vi "constellation_SubVI_-1.vi"(10 "Array":dbl[][](array[numeric]), 11 "N":dbl) -> (3 "Cluster":cluster{dbl[], dbl[]})   [LabVIEW 2014]
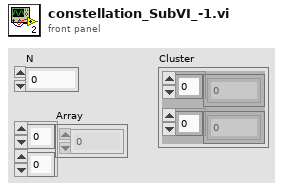
[diagram p1: front panel]
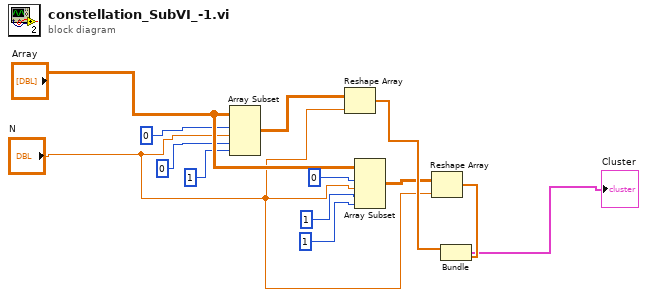
[diagram p0: block diagram]
diagram:
  n1 = Array Subset(array="Array", index (row)=0, length (row)="N", index (col)=0, length (col)=1) -> (w7:dbl[][])
  n2 = Reshape Array(w7, "N") -> (w12:dbl[])
  n3 = Array Subset(array="Array", index (row)=0, length (row)="N", index (col)=1, length (col)=1) -> (w11:dbl[][])
  n4 = Reshape Array(w11, "N") -> (w13:dbl[])
  n5 = Bundle(w12, w13) -> (→"Cluster":cluster{dbl[], dbl[]})  [unwired: 1 in]
